vi "PSK_Packet_Demod.vi"(11 "input waveform":T1={"t0"=0.0, "dt"=1.0, "Y"=[]} caption="waveform" {"Y" format="%.3f"; "dt" format="%^.2e"; "t0" format="%.4f"}) -> (1 "sync found index (symbols)":dbl format="%.4f", 3 "output bit stream":i8[](array[numeric]))   [LabVIEW 2014]
uses:
  <vilib>/addons/Modulation/Analog/controls/Complex Data Waveform.ctl
  <vilib>/addons/Modulation/Digital/General/MT Generate Bits (Galois, PN Order).vi
  <vilib>/addons/Modulation/Digital/Support/Common/Validators/mod_Generate Bits Validate.vi
  <vilib>/addons/Modulation/Analog/support/mod_Set Error Source.vi
  <vilib>/addons/Modulation/Digital/General/MT Generate PSK System Parameters(M).vi
  <vilib>/addons/Modulation/Digital/Support/Common/Validators/mod_Generate Filter Coefficients Validate.vi
  <vilib>/addons/Modulation/Digital/General/subVIs/mod_Generate Filter Coefficients.vi
  <vilib>/addons/Modulation/Digital/General/subVIs/mod_Generate Bits PN Sequence.vi
  <vilib>/addons/Modulation/Digital/General/MT Generate PSK Synchronization Parameters (bit array).vi
  <vilib>/addons/Modulation/niDMT.lvlib
  <vilib>/addons/Modulation/niAMT.lvlib
panel:
  out "Constellation Graph":T2(graph) caption="Tx Signal Constellation"
  in  "filter parameters":T3={"Alpha"=0.5, "Filter Length"=6, "TX Filter"=enum."Root Raised Cos"} {"Alpha" format="%.2f"}
  in  "QPSK System Parameters":T4={"Samples per Symbol"=8, "symbol map"=[], "Differential PSK"=enum."disable", "PSK type"=0} {"PSK type" items=["normal", "shifted", "offset"]; "symbol map" format="%.3f"}
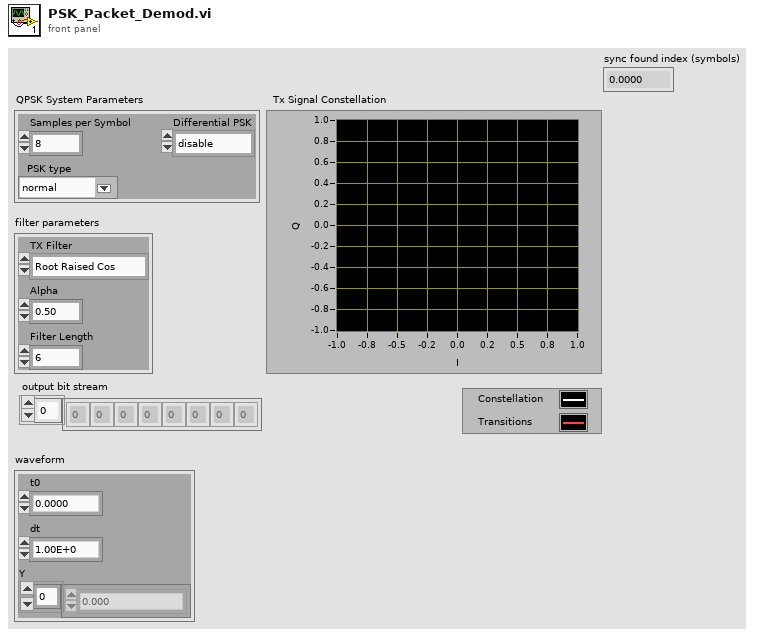
[diagram p1: front panel]
types:
  T1 = typedef "niAMT.lvlib/Complex Data Waveform.ctl" = cluster{"t0":dbl, "dt":dbl, "Y":cdb[]}
  T2 = cluster{"constellation":dbl[], "oversampled data":dbl[]}[]
  T3 = cluster{"Alpha":dbl, "Filter Length":i32, "TX Filter":enum16{"none", "Raised Cosine", "Root Raised Cos", "Gaussian"}}
  T4 = cluster{"Samples per Symbol":i32, "symbol map":cdb[], "Differential PSK":enum16{"disable", "enable"}, "PSK type":u16}
  T5 = enum16{"FSK", "PSK", "QAM", "MSK", "PAM", "ASK", "CPM"}
  T6 = enum16{"none", "Raised Cosine", "Root Raised Cos", "Gaussian"}
  T7 = cluster{"samples per symbol (16)":i32, "symbol map":cdb[], "differential PSK":enum16{"disable", "enable"}, "PSK type":u16}
  T8 = cluster{"expected sync location (symbols)":i32, "sync sequence":cdb[], "sync location uncertainty (symbols)":i32, "sync indent (symbols)":i32}
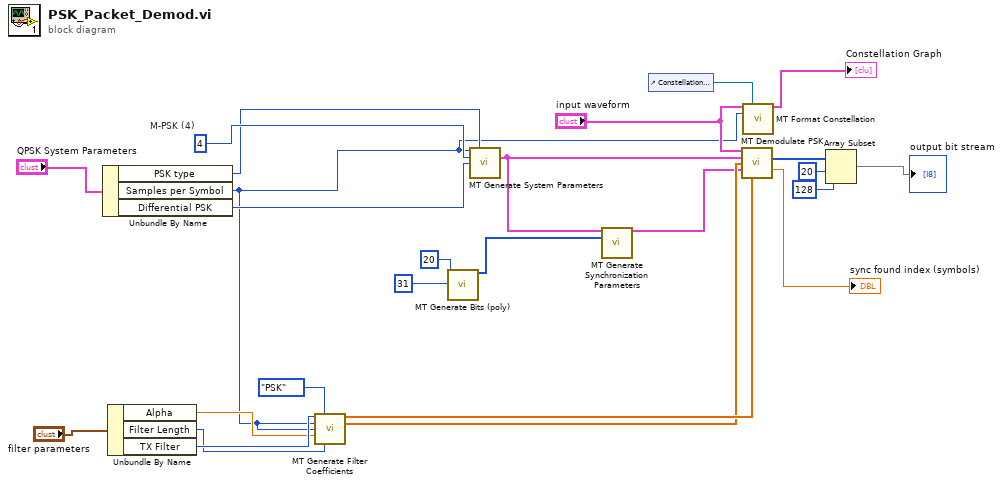
[diagram p0: block diagram]
diagram:
  w18 = 4  # M-PSK (4)
  n1 = Unbundle By Name("QPSK System Parameters") -> ("PSK type"=w17:u16, "Samples per Symbol"=w1:i32, "Differential PSK"=w19:enum16{"disable", "enable"})
  n2 = Unbundle By Name("filter parameters") -> ("Alpha"=w22:dbl, "Filter Length"=w23:i32, "TX Filter"=w24:T6)
  n3 = call <vilib>:"MT Generate Filter Coefficients.vi"("pulse shaping filter (none)"=w24, "modulation type"=T5."PSK", "pulse shaping samples per symbol (16)"=w1, "matched samples per symbol (16)"=w1, "filter parameter"=w22, "filter length (symbols)"=w23) -> ("pulse shaping filter coefficients"=w13:dbl[], "matched filter coefficients"=w12:dbl[])  [unwired: 7 in, 1 out]
  n4 = call-poly <vilib>:"MT Generate Bits (poly).vi"("total bits (128)"=20, "PN sequence order (9)"=31) -> ("output bit stream"=w14:i8[])  [unwired: 11 in, 2 out]
  n5 = call-poly <vilib>:"MT Generate System Parameters.vi"("samples per symbol (16)"=w1, "PSK type"=w17, "M-PSK (4)"=w18, "differential PSK"=w19) -> ("PSK system parameters"=w4:T7)  [unwired: 9 in, 2 out]
  n6 = call-poly <vilib>:"MT Generate Synchronization Parameters.vi"("PSK system parameters"=w4, "sync bits"=w14) -> ("PSK synchronization parameters"=w11:T8)  [unwired: 12 in, 1 out]
  n7 = control-ref of="Constellation Graph"() -> (w6:refnum<vi>)
  n8 = call <vilib>:"MT Demodulate PSK.vi"("input complex waveform"="input waveform", "PSK system parameters"=w4, "matched filter coefficients"=w12, "synchronization parameters"=w11, "pulse shaping filter coefficients"=w13) -> ("output bit stream"=w7:i8[], "sync found index (symbols)"=→"sync found index (symbols)":dbl)  [unwired: 6 in, 3 out]
  n9 = call <vilib>:"MT Format Constellation.vi"("waveform"="input waveform", "constellation reference"=w6, "samples per symbol"=w1) -> ("constellation graph"=→"Constellation Graph":T2)  [unwired: 11 in, 1 out]
  n10 = Array Subset(array=w7, index=20, length=128) -> (→"output bit stream":i8[])
